vi "Configure DC Current.vi"(0 "VISA resource name":refnum<visa-resource-name>, 5 "error in (no error)":errorcluster, 6 "Auto Range? (T: Auto)":bool=TRUE, 7 "Digital Filter (0: Off)":u16(ring) items=["Off", "Moving Filter", "Repeating Filter"], 8 "Custom Range (0 A)":dbl min=0.0 max=10.0 format="%#_6p", 9 "Digital Filter Readings (10)":i32=10, 10 "Function":i32(ring) items=["Primary", "Secondary"], 11 "NPLC":i32(ring)=2 items=["0.001", "0.006", "0.02", "0.06", "0.1", "0.2", "0.6", "1", "2", "10", "100"]) -> (14 "VISA resource name out":refnum<visa-resource-name>, 19 "error out":errorcluster)   [LabVIEW 2020, in "Keithley 2100 Series.lvlib"]
doc: "This VI configures the instrument to measure DC Current."
uses:
  Keithley 2100 Series.lvlib
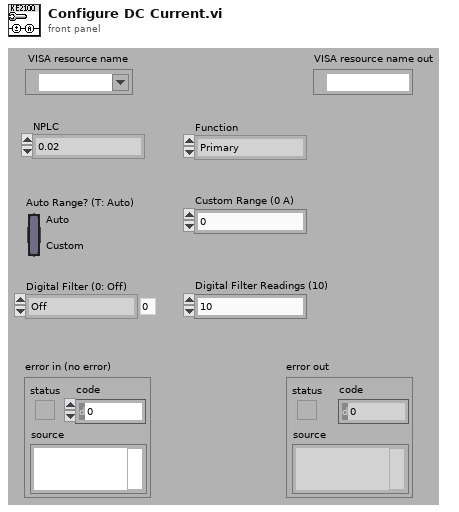
[diagram p1: front panel]
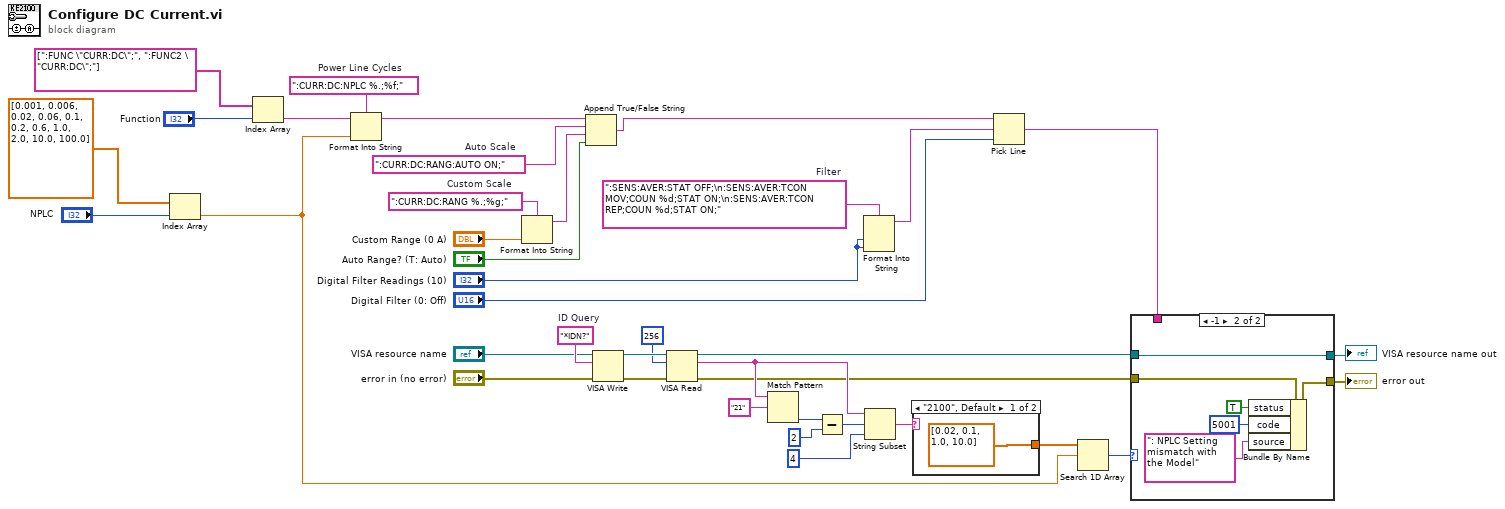
[diagram p0: block diagram]
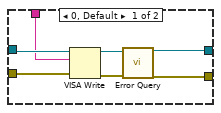
[diagram p2: hidden frame]
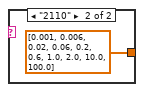
[diagram p3: hidden frame]
diagram:
  w22 = "*IDN?"  # ID Query
  w4 = ":CURR:DC:NPLC %.;%f;"  # Power Line Cycles
  w30 = ":SENS:AVER:STAT OFF;\n:SENS:AVER:TCON MOV;COUN %d;STAT ON;\n:SENS:AVER:TCON REP;COUN %d;STAT ON;"  # Filter
  w33 = ":CURR:DC:RANG:AUTO ON;"  # Auto Scale
  w35 = ":CURR:DC:RANG %.;%g;"  # Custom Scale
  n1 = Index Array(array=dbl[] [0.001, 0.006, 0.02, 0.06, 0.1, 0.2, 0.6, 1.0, 2.0, 10.0, 100.0] ("number"), index="NPLC") -> (element=w12:dbl)
  n2 = Index Array(array=string[] [":FUNC \"CURR:DC\";", ":FUNC2 \"CURR:DC\";"], index="Function") -> (element=w1:string)
  n3 = Format Into String(format string=w4, initial string=w1, w12) -> (resulting string=w37:string)  [unwired: 1 in, 1 out]
  n4 = Format Into String(format string=w35, "Custom Range (0 A)") -> (resulting string=w34:string)  [unwired: 2 in, 1 out]
  n5 = Append True/False String(1:"Auto Range? (T: Auto)", 2:w34, 3:w33, 4:w37) -> (0:w28:string)
  n6 = VISA Write(VISA resource name="VISA resource name", write buffer=w22, error in (no error)="error in (no error)") -> (VISA resource name out=w25:refnum<visa-resource-name>, error out=w24:errorcluster)  [unwired: 1 out]
  n7 = VISA Read(VISA resource name=w25, byte count=u32 256, error in (no error)=w24) -> (VISA resource name out=w9:refnum<visa-resource-name>, read buffer=w14:string, error out=w8:errorcluster)  [unwired: 1 out]
  n8 = Match Pattern(string=w14, regular expression="21") -> (offset past match=w18:i32)  [unwired: 1 in, 3 out]
  n9 = Subtract(x=w18, y=2) -> (x-y=w17:i32)
  n10 = Format Into String(format string=w30, "Digital Filter Readings (10)", "Digital Filter Readings (10)") -> (resulting string=w31:string)  [unwired: 2 in, 1 out]
  n11 = String Subset(string=w14, offset (0)=w17, length (rest)=4 ("length")) -> (substring=w13:string)
  n12 = case shown="\"2100\", Default" w13 {
    tunnel: [dbl[] [0.02, 0.1, 1.0, 10.0] dbl[] [0.001, 0.006, 0.02, 0.06, 0.2, 0.6, 1.0, 2.0, 10.0, 100.0] ("number")] -> w11
    frame "2100", Default {
    }
    frame "2110" {
    }
  }
  n13 = Pick Line(string ("")=w28, multi-line string=w31, line index="Digital Filter (0: Off)") -> (output string=w5:string)
  n14 = Search 1D Array(1D array=w11, element=w12) -> (index of element=w10:i32)  [unwired: 1 in]
  n15 = case shown="-1" w10 {
    tunnel: w9 -> [w45 w53]
    tunnel: w8 -> [w44 w52]
    tunnel: [w43 w53] -> w7
    tunnel: [w42 w50] -> w6
    tunnel: w5 -> [w41 _]
    frame 0, Default {
      n16 = VISA Write(VISA resource name=w45, write buffer=w41, error in (no error)=w44) -> (VISA resource name out=w47:refnum<visa-resource-name>, error out=w46:errorcluster)  [unwired: 1 out]
      n17 = call "Error Query.vi"("VISA resource name"=w47, "error in (no error)"=w46) -> ("VISA resource name out"=w43:refnum<visa-resource-name>, "error out"=w42:errorcluster)  [unwired: 14 in, 2 out]
    }
    frame -1 {
      n18 = Bundle By Name(cluster=w52, "status"=TRUE, "code"=5001, "source"=": NPLC Setting mismatch with the Model") -> (w50:errorcluster)
    }
  }
  "error out" <- w6
  "VISA resource name out" <- w7
